vi "backup_imp_test_v4.vi"() -> ()   [LabVIEW 2014]
uses:
  <vilib>/LabVIEW Targets/FPGA/cRIO/shared/nicrio_ModuleControls/nicrio_cRIO-9237_DataRatesRing.ctl
  <vilib>/LabVIEW Targets/FPGA/cRIO/shared/nicrio_ModuleControls/nicrio_cRIO-9237_ExcitationVoltageRing.ctl
  <vilib>/rvi/FXPMathLib/FxpSinAndCos/subVIs/nifxpmath_SinAndCos_SimConfig.ctl
  <vilib>/rvi/Emulation/niFpgaGetClockAttributes.vi
  <vilib>/rvi/Emulation/niFpgaSctlEmulationGetInTimedLoop.vi
  <vilib>/rvi/Emulation/niFpgaEmulationReportErrorSimple.vi
  <vilib>/rvi/Emulation/niFpgaProcessEmulError.vi
  <vilib>/rvi/interface/RandomDataEmulation/nirviRandomDataMultiElementFPGAFIFO.vi
  <instcachedir>/0/nirviRandomDataMultiElementFPGAFIFO_AD0CFC12EF974623A9C2E4184BC062B2.lvgen/nirviRandomDataMultiElementFPGAFIFO_AD0CFC12EF974623A9C2E4184BC062B2_023.vi
  <vilib>/rvi/interface/RandomDataEmulation/niFpgaRandomDataHandleErrors.vi
  <vilib>/rvi/Emulation/niFpgaCriticalErrorInLSC.vi
  <vilib>/rvi/eio/common/nirviEmuTemplateMethod_errors.vi
  <vilib>/rvi/FXPMathLib/FxpSinAndCos/simVIs/DllFxpSinAndCosTemp_sub.vi
  <vilib>/rvi/eio/common/nirviEmuTemplatePropertySet_errors.vi
  <vilib>/rvi/DataTransferAndStorage/Container/XNode/niFpgaContainer.xnode
  <vilib>/rvi/interface/RandomDataEmulation/nirviRandomDataFpgaMultiElementTemplate.vi
  <vilib>/eio/EIONode/EIONode.xnode
  <vilib>/rvi/FXPMathLib/FxpMul/XNode/nifxpmath_Multiplier.xnode
  <vilib>/rvi/FXPMathLib/FxpSinAndCos/XNode/nifxpmath_SinAndCos.xnode
  <vilib>/rvi/Analysis/measure/butterworth/XNode/niFpgaButterworthFilter.xnode
  <vilib>/rvi/FXPMathLib/FxpSub/XNode/nifxpmath_Sub.xnode
  <vilib>/rvi/FXPMathLib/FxpAdd/XNode/nifxpmath_Add.xnode
  <vilib>/eio/EIOPropertyNode/EIOPropertyNode.xnode
  <vilib>/rvi/eio/common/nirviEmuTemplatePropertyGet_errors.vi
  <vilib>/rvi/eio/common/nirviEmuTemplatePropertyGet_noerrors.vi
  <vilib>/rvi/eio/common/nirviEmuTemplatePropertySet_noerrors.vi
  <vilib>/rvi/FXPMathLib/sim/FxpSim.dll
panel:
  out "Fp_dc":fxp<+/-,32,10>
  out "Fy_dc":fxp<+/-,32,10>
  in  "Zero_y":bool
  in  "Zero_p":bool
  in  "mt0_omega_p":u32
  in  "Encoder reset":bool
  out "fpt_d":fxp<+/-,36,18>
  out "Dp_error_dd":fxp<+/-,36,16>
  out "Dp_error_d":fxp<+/-,33,8>
  in  "Dp_dd coeff.":i32[](array[numeric])=[946630756, 63555534]
  out "Dp_dd":fxp<+/-,36,25>
  out "dFp_PID":fxp<+/-,36,18>
  in  "dFp_PID coeff.":i32[](array[numeric])=[946630756, 63555534]
  out "fpt_i":fxp<+/-,34,18>
  in  "Bv_p":fxp<+/-,22,8>
  in  "Kv_p":fxp<+/-,22,8>
  out "Dp_error":fxp<+/-,22,7>
  out "Dpr_sin":fxp<+/-,22,7>
  in  "Sin offset_p":fxp<+/-,22,7>
  in  "Sin magnitude_p":fxp<+/-,21,6>
  out "Dpr_sin_dd":fxp<+/-,35,20>
  out "Dpr_sin_d":fxp<+/-,33,15>
  out "Sin omega_p":fxp<+/-,34,9>
  in  "Sin wave freq._p (Hz)":fxp<+/-,32,6>
  in  "Dpr_step":fxp<+/-,22,7>
  out "Dpr_for":fxp<+/-,22,7>
  in  "Command_p":i16(ring) items=["Step", "Sine"]
  in  "Ki_p":fxp<+/-,36,9>
  out "Fp_PID":fxp<+/-,36,16>
  in  "fp_tolorance":fxp<+,22,6>
  out "fp_tilde":fxp<+/-,33,10>
  in  "Kd_p":fxp<+/-,36,9>
  in  "Kp_p":fxp<+/-,36,9>
  out "Fr_p":fxp<+/-,32,10>
  in  "S/F coeff_p":fxp<+/-,25,-10>
  in  "S/F coeff_y":fxp<+/-,25,-10>
  out "va_p":fxp<+/-,36,7>
  out "vb_p":fxp<+/-,37,8>
  out "vq_p_F":fxp<+/-,20,5> format="%.57g"
  out "vd_p_F":fxp<+/-,20,5>
  in  "dFp_add":bool
  in  "Stop motor_p":bool
  out "Force_p":fxp<+/-,32,10>
  in  "Strain selection_p":i16(ring) items=["Raw", "Avg.", "Avg. w. filter"]
  out "Strain_p (Avg w. f)":fxp<+/-,36,8>
  in  "Strain_p mean coeff.":i32[](array[numeric])=[946630756, 63555534]
  out "Strain_p (Avg)":fxp<+/-,32,4>
  out "Raw Strain_p":fxp<+/-,36,4>
  out "Mod6/AI3":fxp<+/-,32,4>
  in  "Strain gage reset_p":bool
  out "Dp_d (mm/s)":fxp<+/-,36,11>
  out "omega_p (rad/s)":fxp<+/-,20,9>
  out "mt_omega_p":u32
  out "rad_p(NrTheta)":fxp<+/-,33,20>
  out "D_p(mm)":fxp<+/-,32,7>
  out "Encoder Position_p":i32
  in  "Encoder reset_p":bool
  out "Strain_y (Avg w. f)":fxp<+/-,36,8>
  in  "Strain_y mean coeff.":i32[](array[numeric])=[-898916953, 1957103773, 3888751]
  out "Dyr_for":fxp<+/-,22,7>
  in  "Command_y":i16(ring) items=["Step", "Sine"]
  out "Strain_y (Avg)":fxp<+/-,32,4>
  in  "Strain selection_y":i16(ring) items=["Raw", "Avg.", "Avg. w. filter"]
  out "vb_y":fxp<+/-,38,8>
  out "va_y":fxp<+/-,38,8>
  out "fyt_d":fxp<+/-,36,18>
  out "Fr_y":fxp<+/-,32,10>
  in  "Bv_y":fxp<+/-,22,8>
  out "Dy_error_dd":fxp<+/-,36,16>
  out "Dy_error_d":fxp<+/-,33,8>
  in  "Kv_y":fxp<+/-,22,8>
  out "Dy_error":fxp<+/-,22,7>
  out "Dyr_sin_dd":fxp<+/-,35,20>
  out "Dyr_sin_d":fxp<+/-,33,15>
  out "Sin omega_y":fxp<+/-,34,9>
  out "Dyr_sin":fxp<+/-,22,7>
  in  "Sin offset_y":fxp<+/-,22,7>
  in  "Sin magnitude_y":fxp<+/-,21,6>
  out "Time now(s)":fxp<+,52,14>
  in  "Sin wave freq._y (Hz)":fxp<+/-,32,6>
  in  "Dyr_step":fxp<+/-,22,7>
  in  "Drive mode":i16(ring) items=["Backward", "Forward"]
  out "Dy_dd":fxp<+/-,36,25>
  in  "Dy_dd coeff.":i32[](array[numeric])=[946630756, 63555534]
  out "dFy_PID":fxp<+/-,36,18>
  in  "dFy_PID coeff.":i32[](array[numeric])=[946630756, 63555534]
  out "fyt_i":fxp<+/-,36,16>
  out "Fy_PID":fxp<+/-,36,16>
  in  "fy_tolorance":fxp<+,22,6>
  in  "Ki_y":fxp<+/-,36,9>
  in  "Kd_y":fxp<+/-,36,9>
  out "fy_tilde":fxp<+/-,32,10>
  in  "Kp_y":fxp<+/-,36,9>
  out "vq_y_F":fxp<+/-,20,5> format="%.57g"
  out "vd_y_F":fxp<+/-,20,5>
  in  "dFy_add":bool
  in  "Stop motor_y":bool
  out "Dy_d (mm/s)":fxp<+/-,36,11>
  out "omega_y (rad/s)":fxp<+/-,20,9>
  in  "mt0_omega_y":u32
  out "mt_omega_y":u32
  out "rad_y(NrTheta)":fxp<+/-,33,20>
  out "D_y(mm)":fxp<+/-,32,7>
  out "Encoder Position_y":i32
  in  "Encoder reset_y":bool
  in  "Ini coe.":bool
  out "Loop rate (kHz)":fxp<+/-,36,7>
  out "Force_y":fxp<+/-,32,10>
  out "Raw Strain_y":fxp<+/-,36,4>
  in  "Strain gage reset_y":bool
  in  "Stop (Strain)":bool
  out "Mod6/AI2":fxp<+/-,32,4>
  in  "Excitation Voltage":T1 items=["2.5 Volts", "3.3 Volts", "5.0 Volts", "10.0 Volts", "External Excitation"]
  in  "Data Rate":T2=1 items=["50.000 kS/s (NI 9237)"=1, "25.000 kS/s (NI 9237)"=2, "16.667 kS/s (NI 9237)"=3, "12.500 kS/s (NI 9237)"=4, "10.000 kS/s (NI 9237)"=5, "8.333 kS/s (NI 9237)"=6, "7.143 kS/s (NI 9237)"=7, "6.250 kS/s (NI 9237)"=8, "5.556 kS/s (NI 9237)"=9, "5.000 kS/s (NI 9237)"=10, "4.545 kS/s (NI 9237)"=11, "4.167 kS/s (NI 9237)"=12, "3.846 kS/s (NI 9237)"=13, "3.571 kS/s (NI 9237)"=14, "3.333 kS/s (NI 9237)"=15, "3.125 kS/s (NI 9237)"=16, "2.941 kS/s (NI 9237)"=17, "2.778 kS/s (NI 9237)"=18, "2.632 kS/s (NI 9237)"=19, "2.500 kS/s (NI 9237)"=20, "2.381 kS/s (NI 9237)"=21, "2.273 kS/s (NI 9237)"=22, "2.174 kS/s (NI 9237)"=23, "2.083 kS/s (NI 9237)"=24, "2.000 kS/s (NI 9237)"=25, "1.923 kS/s (NI 9237)"=26, "1.852 kS/s (NI 9237)"=27, "1.786 kS/s (NI 9237)"=28, "1.724 kS/s (NI 9237)"=29, "1.667 kS/s (NI 9237)"=30, "1.613 kS/s (NI 9237)"=31]
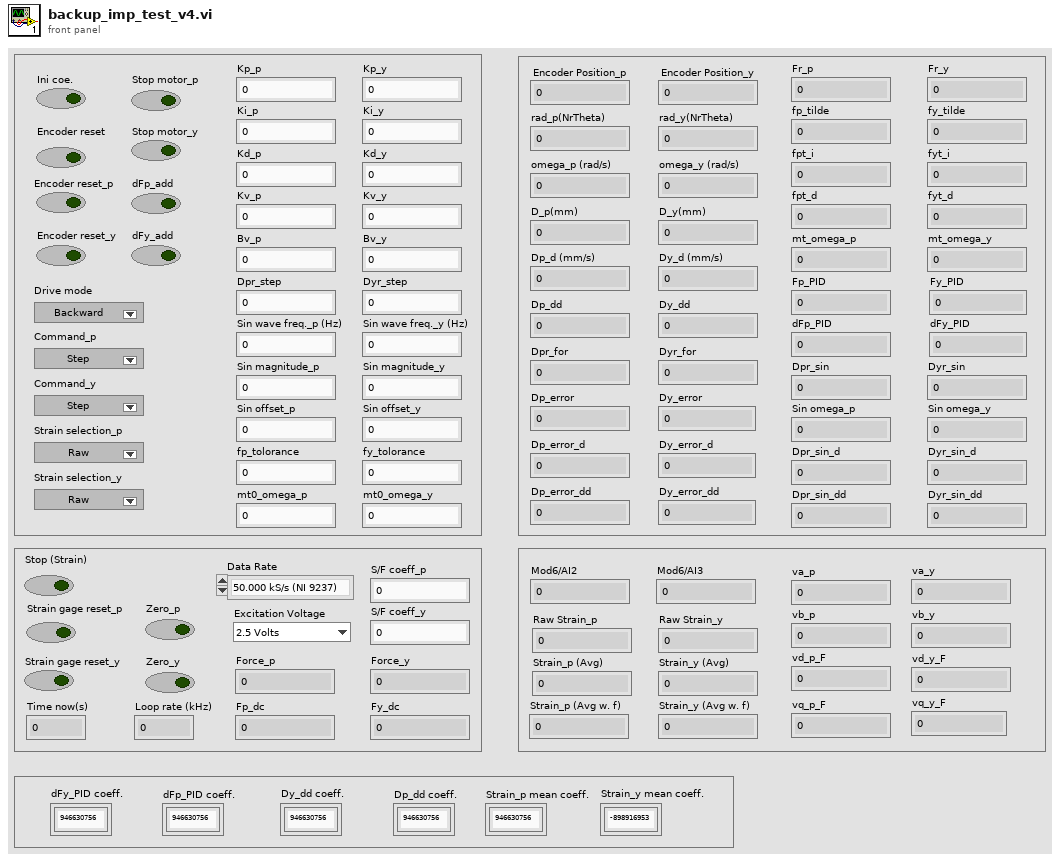
[diagram p1: front panel]
types:
  T1 = typedef "nicrio_cRIO-9237_ExcitationVoltageRing.ctl" = u8
  T2 = typedef "nicrio_cRIO-9237_DataRatesRing.ctl" = u8
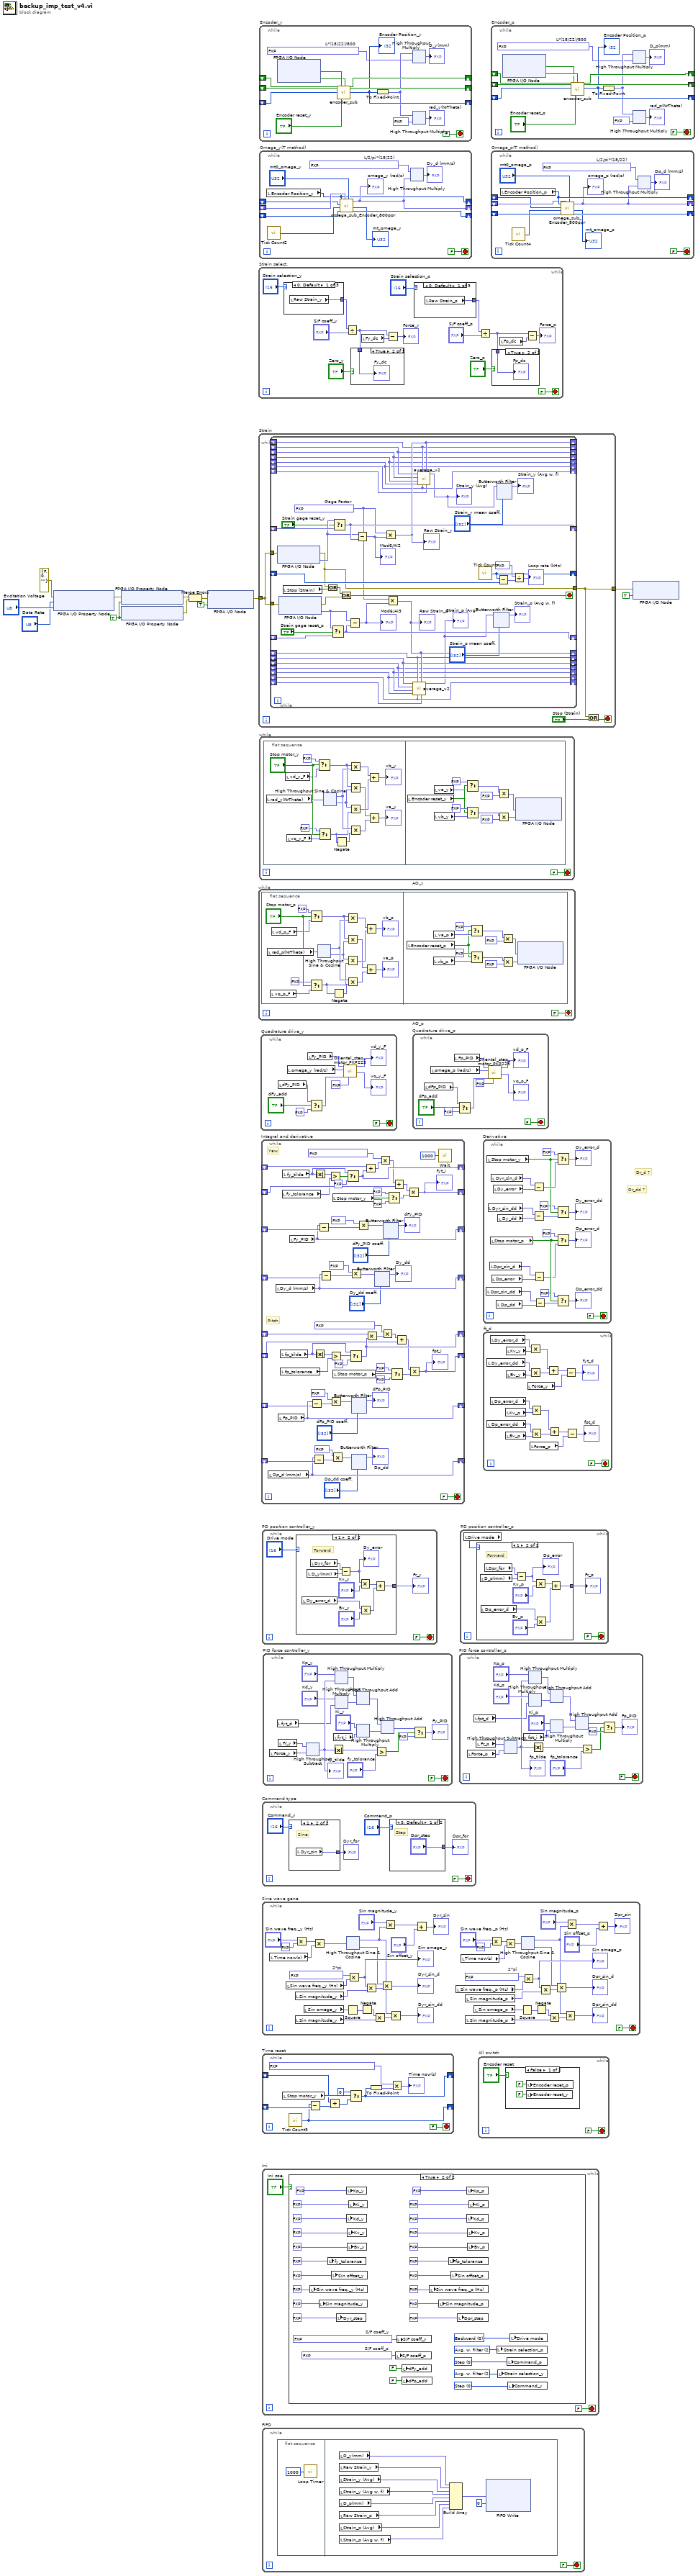
[diagram p0: block diagram]
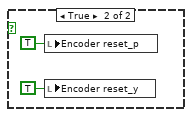
[diagram p2: hidden frame]
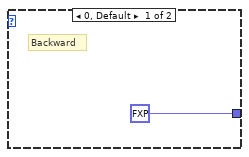
[diagram p3: hidden frame]
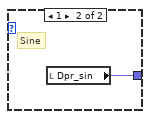
[diagram p4: hidden frame]
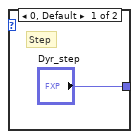
[diagram p5: hidden frame]
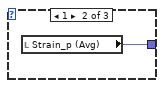
[diagram p8: hidden frame]
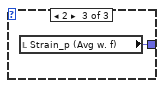
[diagram p9: hidden frame]
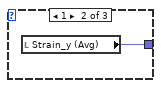
[diagram p10: hidden frame]
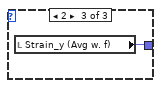
[diagram p11: hidden frame]
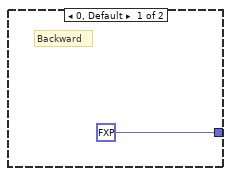
[diagram p12: hidden frame]
diagram:
  w5 = TRUE ("Half-Bridge Enable")
  # "Dr_dd ?"
  # "Dr_d ?"
  n1 = xnode "FPGA I/O Property Node"("error in"=errorcluster {"status"=FALSE, "code"=0, "source"=""}, "Data Rate"="Data Rate", "Excitation Voltage"="Excitation Voltage") -> ("error out"=w10:errorcluster)  [unwired: 1 in, 1 out]
  n2 = xnode "FPGA I/O Property Node"("error in"=w10, "Half-Bridge Enable"=w5) -> ("error out"=w3:errorcluster)  [unwired: 1 in, 1 out]
  n3 = xnode "FPGA I/O Property Node"("Half-Bridge Enable"=w5) -> ("error out"=w2:errorcluster)  [unwired: 2 in, 1 out]
  n4 = Merge Errors(w3, w2) -> (w4:errorcluster)
  n5 = xnode "FPGA I/O Node"("error in"=w4, "Mod6/Start"=TRUE) -> ("error out"=w8:errorcluster)  [unwired: 1 in, 1 out]
  n6 = while "Strain select." {
    stop <- FALSE stop-if-true
    n7 = case shown="0, Default" "Strain selection_y" {
      tunnel: [w33 w34 w35] -> w26
      frame 0, Default {
        n8 = local read "Raw Strain_y"() -> (w33:fxp<+/-,36,4>)
      }
      frame 1 {
        n9 = local read "Strain_y (Avg)"() -> (w34:fxp<+/-,32,4>)
      }
      frame 2 {
        n10 = local read "Strain_y (Avg w. f)"() -> (w35:fxp<+/-,36,8>)
      }
    }
    n11 = Divide(x=w26, y="S/F coeff_y") -> (x/y=w19:fxp<+/-,32,10>)
    n12 = case shown="True" "Zero_y" {
      tunnel: w19 -> [_ w29]
      frame False {
      }
      frame True {
        "Fy_dc" <- w29
      }
    }
    n13 = local read "Fy_dc"() -> (w20:fxp<+/-,32,10>)
    n14 = Subtract(x=w19, y=w20) -> (x-y=→"Force_y":fxp<+/-,33,11>)
    n15 = case shown="0, Default" "Strain selection_p" {
      tunnel: [w30 w31 w32] -> w24
      frame 0, Default {
        n16 = local read "Raw Strain_p"() -> (w30:fxp<+/-,36,4>)
      }
      frame 1 {
        n17 = local read "Strain_p (Avg)"() -> (w31:fxp<+/-,32,4>)
      }
      frame 2 {
        n18 = local read "Strain_p (Avg w. f)"() -> (w32:fxp<+/-,36,8>)
      }
    }
    n19 = Divide(x=w24, y="S/F coeff_p") -> (x/y=w16:fxp<+/-,32,10>)
    n20 = case shown="True" "Zero_p" {
      tunnel: w16 -> [_ w28]
      frame False {
      }
      frame True {
        "Fp_dc" <- w28
      }
    }
    n21 = local read "Fp_dc"() -> (w14:fxp<+/-,32,10>)
    n22 = Subtract(x=w16, y=w14) -> (x-y=→"Force_p":fxp<+/-,33,11>)
  }
  n23 = while "Strain" {
    tunnel: w8 -> [w38]
    tunnel: [w36] -> w1
    stop <- w37 stop-if-true
    n24 = while {
      tunnel: w38 -> [w84]
      tunnel: [w57] -> w36
      shift-right: [w81] -> _
      shift-left: _ -> [w82]
      shift-right: [w77] -> _
      shift-left: _ -> [w78]
      shift-right: [w72] -> _
      shift-left: _ -> [w71]
      shift-right: [w71] -> _
      shift-left: _ -> [w70]
      shift-right: [w70] -> _
      shift-left: _ -> [w69]
      shift-right: [w69] -> _
      shift-left: _ -> [w68]
      shift-right: [w68] -> _
      shift-left: _ -> [w67]
      shift-right: [w67] -> _
      shift-left: _ -> [w66]
      shift-right: [w66] -> _
      shift-left: _ -> [w65]
      tunnel: w38 -> [w61]
      shift-right: [w54] -> _
      shift-left: _ -> [w55]
      shift-right: [w50] -> _
      shift-left: _ -> [w49]
      shift-right: [w49] -> _
      shift-left: _ -> [w48]
      shift-right: [w48] -> _
      shift-left: _ -> [w47]
      shift-right: [w47] -> _
      shift-left: _ -> [w46]
      shift-right: [w46] -> _
      shift-left: _ -> [w45]
      shift-right: [w45] -> _
      shift-left: _ -> [w44]
      shift-right: [w44] -> _
      shift-left: _ -> [w43]
      stop <- w58 stop-if-true
      w52 = fxp<+,20,2> 2.115001678466797  # Gage Factor
      n25 = xnode "FPGA I/O Node"("error in"=w84) -> ("error out"=w57:errorcluster, "Mod6/AI2"=w79:fxp<+/-,24,-4>)  [unwired: 1 in, 1 out]
      n26 = xnode "FPGA I/O Node"("error in"=w61) -> ("error out"=w59:errorcluster, "Mod6/AI3"=w53:fxp<+/-,24,-4>)  [unwired: 1 in, 1 out]
      n27 = local read "Stop (Strain)"() -> (w83:bool)
      n28 = Or(x=w57, y=w83) -> (x .or. y?=w60:bool)
      n29 = Select(t=w53, s="Strain gage reset_p", f=w55) -> (s? t:f=w54:fxp<+/-,24,-4>)
      n30 = Select(t=w79, s="Strain gage reset_y", f=w82) -> (s? t:f=w81:fxp<+/-,24,-4>)
      n31 = Or(x=w60, y=w59) -> (x .or. y?=w58:bool)
      n32 = Subtract(x=w53, y=w54) -> (x-y=w51:fxp<+/-,25,-3>)
      "Mod6/AI3" <- w51
      n33 = Subtract(x=w79, y=w81) -> (x-y=w80:fxp<+/-,25,-3>)
      "Mod6/AI2" <- w80
      n34 = Multiply(x=w52, y=w80) -> (x*y=w72:fxp<+/-,41,6>)
      "Raw Strain_y" <- w72
      n35 = Multiply(x=w52, y=w51) -> (x*y=w50:fxp<+/-,45,-1>)
      "Raw Strain_p" <- w50
      n36 = call "average_v2.vi"("Numeric 8"=w43, "Numeric"=w50, "Numeric 7"=w44, "Numeric 2"=w49, "Numeric 6"=w45, "Numeric 5"=w46, "Numeric 4"=w47, "Numeric 3"=w48) -> ("Mean (8pt)"=w42:fxp<+/-,32,4>)  [unwired: 1 in, 2 out]
      "Strain_p (Avg)" <- w42
      n37 = call "average_v2.vi"("Numeric 8"=w65, "Numeric"=w72, "Numeric 7"=w66, "Numeric 2"=w71, "Numeric 6"=w67, "Numeric 5"=w68, "Numeric 4"=w69, "Numeric 3"=w70) -> ("Mean (8pt)"=w64:fxp<+/-,32,4>)  [unwired: 1 in, 2 out]
      "Strain_y (Avg)" <- w64
      n38 = call "Tick Count"() -> ("Tick Count(uSec)"=w77:u32)
      n39 = xnode "Butterworth Filter"("input data"=w42, "scaled coefficients"="Strain_p mean coeff.") -> ("output data"=→"Strain_p (Avg w. f)":fxp<+/-,36,8>)  [unwired: 1 in]
      n40 = xnode "Butterworth Filter"("input data"=w64, "scaled coefficients"="Strain_y mean coeff.") -> ("output data"=→"Strain_y (Avg w. f)":fxp<+/-,32,4>)  [unwired: 1 in]
      n41 = Subtract(x=w77, y=w78) -> (x-y=w75:fxp<+/-,32,16>)
      n42 = Divide(x=fxp<+,7,10> 1000.0, y=w75) -> (x/y=→"Loop rate (kHz)":fxp<+/-,40,27>)
    }
    n43 = Or(x=w36, y="Stop (Strain)") -> (x .or. y?=w37:bool)
  }
  n44 = while "AO_p" {
    stop <- FALSE stop-if-true
    n45 = flat-sequence {
      frame #0 {
        n46 = local read "rad_p(NrTheta)"() -> (w113:fxp<+/-,33,20>)
        n47 = local read "vq_p_F"() -> (w114:fxp<+/-,20,5>)
        n48 = local read "vd_p_F"() -> (w116:fxp<+/-,20,5>)
        n49 = Select(t=fxp<+/-,20,5> 0.0, s="Stop motor_p", f=w116) -> (s? t:f=w105:fxp<+/-,20,5>)
        n50 = Select(t=fxp<+,1,1> 0.0, s="Stop motor_p", f=w114) -> (s? t:f=w104:fxp<+/-,20,5>)
        n51 = xnode "High Throughput Sine & Cosine"("x (pi)"=w113) -> ("sin(x)"=w107:fxp<+/-,16,2>, "cos(x)"=w106:fxp<+/-,16,2>)
        n52 = Negate(x=w104) -> (-x=w112:fxp<+/-,21,6>)
        n53 = Multiply(x=w105, y=w107) -> (x*y=w111:fxp<+/-,36,7>)
        n54 = Multiply(x=w105, y=w106) -> (x*y=w109:fxp<+/-,36,7>)
        n55 = Multiply(x=w106, y=w104) -> (x*y=w110:fxp<+/-,36,7>)
        n56 = Multiply(x=w107, y=w112) -> (x*y=w108:fxp<+/-,35,6>)
        n57 = Add(x=w111, y=w110) -> (x+y=→"vb_p":fxp<+/-,37,8>)
        n58 = Add(x=w109, y=w108) -> (x+y=→"va_p":fxp<+/-,36,7>)
      }
      frame #1 {
        n59 = local read "Encoder reset_p"() -> (w149:bool)
        n60 = local read "vb_p"() -> (w150:fxp<+/-,37,8>)
        n61 = local read "va_p"() -> (w151:fxp<+/-,36,7>)
        n62 = Select(t=fxp<+,2,2> 3.0, s=w149, f=w151) -> (s? t:f=w157:fxp<+/-,36,7>)
        n63 = Select(t=fxp<+,1,1> 0.0, s=w149, f=w150) -> (s? t:f=w156:fxp<+/-,37,8>)
        n64 = Multiply(x=w157, y=fxp<+/-,1,0> -0.5) -> (x*y=w152:fxp<+/-,36,6>)
        n65 = Multiply(x=w156, y=fxp<+/-,1,0> -0.5) -> (x*y=w153:fxp<+/-,36,6>)
        n66 = xnode "FPGA I/O Node"("Mod8/AO0"=w152, "Mod8/AO1"=w153) -> ()  [unwired: 2 in, 2 out]
      }
    }
  }
  n67 = while "AO_y" {
    stop <- FALSE stop-if-true
    n68 = flat-sequence {
      frame #0 {
        n69 = local read "rad_y(NrTheta)"() -> (w177:fxp<+/-,33,20>)
        n70 = local read "vd_y_F"() -> (w175:fxp<+/-,20,5>)
        n71 = local read "vq_y_F"() -> (w174:fxp<+/-,20,5>)
        n72 = Select(t=fxp<+/-,20,5> 0.0, s="Stop motor_y", f=w175) -> (s? t:f=w169:fxp<+/-,20,5>)
        n73 = Select(t=fxp<+/-,20,5> 0.0, s="Stop motor_y", f=w174) -> (s? t:f=w168:fxp<+/-,20,5>)
        n74 = xnode "High Throughput Sine & Cosine"("x (pi)"=w177) -> ("sin(x)"=w171:fxp<+/-,17,2>, "cos(x)"=w170:fxp<+/-,17,2>)
        n75 = Negate(x=w168) -> (-x=w167:fxp<+/-,21,6>)
        n76 = Multiply(x=w169, y=w171) -> (x*y=w166:fxp<+/-,37,7>)
        n77 = Multiply(x=w169, y=w170) -> (x*y=w164:fxp<+/-,37,7>)
        n78 = Multiply(x=w170, y=w168) -> (x*y=w165:fxp<+/-,37,7>)
        n79 = Multiply(x=w171, y=w167) -> (x*y=w163:fxp<+/-,36,6>)
        n80 = Add(x=w166, y=w165) -> (x+y=→"vb_y":fxp<+/-,38,8>)
        n81 = Add(x=w164, y=w163) -> (x+y=→"va_y":fxp<+/-,37,7>)
      }
      frame #1 {
        n82 = local read "Encoder reset_y"() -> (w210:bool)
        n83 = local read "va_y"() -> (w209:fxp<+/-,38,8>)
        n84 = local read "vb_y"() -> (w208:fxp<+/-,38,8>)
        n85 = Select(t=fxp<+,2,2> 3.0, s=w210, f=w209) -> (s? t:f=w214:fxp<+/-,38,8>)
        n86 = Select(t=fxp<+,1,1> 0.0, s=w210, f=w208) -> (s? t:f=w213:fxp<+/-,38,8>)
        n87 = Multiply(x=w214, y=fxp<+/-,1,0> -0.5) -> (x*y=w217:fxp<+/-,39,8>)
        n88 = Multiply(x=w213, y=fxp<+/-,1,0> -0.5) -> (x*y=w218:fxp<+/-,37,6>)
        n89 = xnode "FPGA I/O Node"("Mod8/AO2"=w217, "Mod8/AO3"=w218) -> ()  [unwired: 2 in, 2 out]
      }
    }
  }
  n90 = while "Encoder_y" {
    shift-right: [w230] -> _
    shift-left: _ -> [w231]
    shift-right: [w232] -> _
    shift-left: _ -> [w233]
    shift-right: [w225] -> _
    shift-left: _ -> [w229]
    stop <- FALSE stop-if-true
    w222 = fxp<+/-,32,0> 0.0020454544574022293  # L*(18/22)/800
    n91 = xnode "FPGA I/O Node"() -> ("Mod4/DI3"=w228:bool, "Mod4/DI4"=w227:bool)  [unwired: 2 in, 2 out]
    n92 = call "encoder_sub.vi"("A_pre"=w231, "B_pre"=w233, "Encoder Position_pre"=w229, "A input"=w228, "Encoder Position Reset"="Encoder reset_y", "B input"=w227) -> ("A"=w230:bool, "B"=w232:bool, "Encoder Position (Counts)"=w225:i32)  [unwired: 19 in]
    "Encoder Position_y" <- w225
    n93 = To Fixed-Point(number=w225) -> (fixed-point=w224:fxp<+/-,32,32>)  [unwired: 1 in]
    n94 = xnode ("High Throughput Multiply")("x"=w224, "y"=w222) -> ("x*y"=→"D_y(mm)":fxp<+/-,64,32>)
    n95 = xnode ("High Throughput Multiply")("x"=w224, "y"=fxp<+/-,16,1> 0.125) -> ("x*y"=→"rad_y(NrTheta)":fxp<+/-,48,33>)
  }
  n96 = while "Omega_y(T method)" {
    shift-right: [w235] -> _
    shift-left: _ -> [w236]
    shift-right: [w239] -> _
    shift-left: _ -> [w241]
    shift-right: [w243] -> _
    shift-left: _ -> [w244]
    stop <- FALSE stop-if-true
    w238 = fxp<+/-,32,0> 0.2604353614151478  # L/2/pi*(18/22)
    n97 = local read "Encoder Position_y"() -> (w235:i32)
    n98 = call "Tick Count2"() -> ("Tick Count(Ticks)"=w245:u32)
    n99 = call "omega_sub_Encoder_800ppr.vi"("mt0"="mt0_omega_y", "omega_pre"=w241, "ticks_m_pre"=w244, "ticks"=w245, "count_pre"=w236, "count"=w235) -> ("ticks_m"=w243:u32, "mt"=→"mt_omega_y":u32, "omega"=w239:fxp<+/-,36,13>)  [unwired: 3 in]
    "omega_y (rad/s)" <- w239
    n100 = xnode ("High Throughput Multiply")("x"=w238, "y"=w239) -> ("x*y"=→"Dy_d (mm/s)":fxp<+/-,64,13>)
  }
  n101 = while "Quadrature drive_y" {
    stop <- FALSE stop-if-true
    n102 = local read "dFy_PID"() -> (w247:fxp<+/-,36,18>)
    n103 = local read "omega_y (rad/s)"() -> (w255:fxp<+/-,20,9>)
    n104 = local read "Fy_PID"() -> (w248:fxp<+/-,36,16>)
    n105 = Select(t=w247, s="dFy_add", f=fxp<+,1,1> 0.0) -> (s? t:f=w251:fxp<+/-,36,18>)
    n106 = call "Oriental_step_motor_PKP225.vi"("F_Threshold"=fxp<+,12,12> 10.0, "dFmr"=w251, "omega"=w255, "Fmr"=w248) -> ("vq_F"=→"vq_y_F":fxp<+/-,20,5>, "vd_F"=→"vd_y_F":fxp<+/-,20,5>)  [unwired: 6 in]
  }
  n107 = while "Integral and derivative" {
    shift-right: [w311] -> _
    shift-left: _ -> [w310]
    shift-right: [w303] -> _
    shift-left: _ -> [w302]
    shift-right: [w313] -> _
    shift-left: _ -> [w314]
    shift-right: [w293] -> _
    shift-left: _ -> [w292]
    shift-right: [w279] -> _
    shift-left: _ -> [w282]
    shift-right: [w272] -> _
    shift-left: _ -> [w271]
    shift-right: [w266] -> _
    shift-left: _ -> [w265]
    shift-right: [w261] -> _
    shift-left: _ -> [w262]
    stop <- FALSE stop-if-true
    # "Pitch"
    # "Yaw"
    n108 = local read "Dp_d (mm/s)"() -> (w261:fxp<+/-,36,11>)
    n109 = local read "Dy_d (mm/s)"() -> (w293:fxp<+/-,36,11>)
    n110 = local read "Fp_PID"() -> (w266:fxp<+/-,36,16>)
    n111 = local read "fp_tilde"() -> (w283:fxp<+/-,33,10>)
    n112 = local read "fp_tolorance"() -> (w286:fxp<+,22,6>)
    n113 = local read "fy_tolorance"() -> (w289:fxp<+,22,6>)
    n114 = local read "fy_tilde"() -> (w315:fxp<+/-,32,10>)
    n115 = local read "Fy_PID"() -> (w313:fxp<+/-,36,16>)
    n116 = Subtract(x=w266, y=w265) -> (x-y=w270:fxp<+/-,37,17>)
    n117 = Subtract(x=w261, y=w262) -> (x-y=w263:fxp<+/-,37,12>)
    n118 = Absolute Value(x=w283) -> (abs(x)=w287:fxp<+,33,10>)
    n119 = Absolute Value(x=w315) -> (abs(x)=w317:fxp<+,32,10>)
    n120 = Subtract(x=w313, y=w314) -> (x-y=w301:fxp<+/-,37,17>)
    n121 = Subtract(x=w293, y=w292) -> (x-y=w295:fxp<+/-,36,11>)
    n122 = Greater?(x=w317, y=w289) -> (0:w318:bool)
    n123 = Greater?(x=w287, y=w286) -> (0:w285:bool)
    n124 = Multiply(x=fxp<+,7,10> 1000.0, y=w270) -> (x*y=w268:fxp<+/-,32,18>)
    n125 = Multiply(x=fxp<+,7,10> 1000.0, y=w263) -> (x*y=w259:fxp<+/-,36,21>)
    n126 = local read "Stop motor_y"() -> (w304:bool)
    n127 = local read "Stop motor_p"() -> (w274:bool)
    n128 = Select(t=w315, s=w318, f=fxp<+/-,33,11> 0.0) -> (s? t:f=w311:fxp<+/-,33,11>)
    n129 = Select(t=w283, s=w285, f=fxp<+,1,1> 0.0) -> (s? t:f=w279:fxp<+/-,33,10>)
    n130 = Multiply(x=fxp<+,7,10> 1000.0, y=w295) -> (x*y=w294:fxp<+/-,36,21>)
    n131 = xnode "Butterworth Filter"("input data"=w268, "scaled coefficients"="dFp_PID coeff.") -> ("output data"=→"dFp_PID":fxp<+/-,36,22>)  [unwired: 1 in]
    n132 = xnode "Butterworth Filter"("input data"=w259, "scaled coefficients"="Dp_dd coeff.") -> ("output data"=→"Dp_dd":fxp<+/-,36,25>)  [unwired: 1 in]
    n133 = Multiply(x=fxp<+,7,10> 1000.0, y=w301) -> (x*y=w298:fxp<+/-,32,18>)
    n134 = Add(x=w310, y=w311) -> (x+y=w316:fxp<+/-,34,12>)
    n135 = Multiply(x=w282, y=w279) -> (x*y=w281:fxp<+/-,34,12>)
    n136 = xnode "Butterworth Filter"("input data"=w294, "scaled coefficients"="Dy_dd coeff.") -> ("output data"=→"Dy_dd":fxp<+/-,36,25>)  [unwired: 1 in]
    n137 = Multiply(x=fxp<+/-,30,12> 0.000499725341796875, y=w316) -> (x*y=w309:fxp<+/-,34,10>)
    n138 = Multiply(x=fxp<+/-,30,12> 0.000499725341796875, y=w281) -> (x*y=w278:fxp<+/-,34,10>)
    n139 = xnode "Butterworth Filter"("input data"=w298, "scaled coefficients"="dFy_PID coeff.") -> ("output data"=→"dFy_PID":fxp<+/-,36,22>)  [unwired: 1 in]
    n140 = Select(t=fxp<+,1,1> 0.0, s=w304, f=fxp<+,1,1> 1.0) -> (s? t:f=w307:fxp<+,1,1>)
    n141 = Select(t=fxp<+,1,1> 0.0, s=w274, f=fxp<+,1,1> 1.0) -> (s? t:f=w276:fxp<+,1,1>)
    n142 = Add(x=w309, y=w302) -> (x+y=w308:fxp<+/-,36,16>)
    n143 = Add(x=w278, y=w271) -> (x+y=w277:fxp<+/-,36,16>)
    n144 = Multiply(x=w308, y=w307) -> (x*y=w303:fxp<+/-,34,18>)
    "fyt_i" <- w303
    n145 = Multiply(x=w277, y=w276) -> (x*y=w272:fxp<+/-,34,18>)
    "fpt_i" <- w272
    n146 = call "Wait"("Count(uSec)"=u32 1000) -> ()  [unwired: 1 out]
  }
  n147 = while "PD position controller_y" {
    stop <- FALSE stop-if-true
    n148 = case shown="1" "Drive mode" {
      tunnel: [fxp<+/-,62,19> 0.0 w357] -> w353
      frame 0, Default {
        # "Backward"
      }
      frame 1 {
        # "Forward"
        n149 = local read "Dy_error_d"() -> (w359:fxp<+/-,33,8>)
        n150 = local read "D_y(mm)"() -> (w364:fxp<+/-,32,7>)
        n151 = local read "Dyr_for"() -> (w356:fxp<+/-,22,7>)
        n152 = Subtract(x=w356, y=w364) -> (x-y=w363:fxp<+/-,33,8>)
        "Dy_error" <- w363
        n153 = Multiply(x=w363, y="Kv_y") -> (x*y=w361:fxp<+/-,54,15>)
        n154 = Multiply(x=w359, y="Bv_y") -> (x*y=w358:fxp<+/-,55,16>)
        n155 = Add(x=w361, y=w358) -> (x+y=w357:fxp<+/-,55,16>)
      }
    }
    "Fr_y" <- w353
  }
  n156 = while "Command type" {
    stop <- FALSE stop-if-true
    n157 = case shown="1" "Command_y" {
      tunnel: ["Dyr_step" w373] -> w368
      frame 0, Default {
        # "Step"
      }
      frame 1 {
        # "Sine"
        n158 = local read "Dyr_sin"() -> (w373:fxp<+/-,22,7>)
      }
    }
    "Dyr_for" <- w368
    n159 = case shown="0, Default" "Command_p" {
      tunnel: ["Dpr_step" w371] -> w366
      frame 0, Default {
        # "Step"
      }
      frame 1 {
        # "Sine"
        n160 = local read "Dpr_sin"() -> (w371:fxp<+/-,22,7>)
      }
    }
    "Dpr_for" <- w366
  }
  n161 = while "Sine wave gene" {
    stop <- FALSE stop-if-true
    w379 = fxp<+,20,3> 6.2831878662109375  # 2*pi
    w411 = fxp<+,20,3> 6.2831878662109375  # 2*pi
    n162 = local read "Time now(s)"() -> (w417:fxp<+,52,14>)
    n163 = local read "Sin wave freq._y (Hz)"() -> (w410:fxp<+/-,32,6>)
    n164 = Multiply(x="Sin wave freq._y (Hz)", y=fxp<+/-,10,3> 2.0) -> (x*y=w418:fxp<+/-,41,9>)
    n165 = local read "Sin magnitude_y"() -> (w408:fxp<+/-,21,6>)
    n166 = local read "Sin magnitude_y"() -> (w401:fxp<+/-,21,6>)
    n167 = local read "Sin omega_y"() -> (w404:fxp<+/-,34,9>)
    n168 = Multiply(x=w418, y=w417) -> (x*y=w416:fxp<+/-,41,19>)
    n169 = Square(x=w404) -> (x^2=w403:fxp<+,34,18>)
    n170 = xnode "High Throughput Sine & Cosine"("x (pi)"=w416) -> ("sin(x)"=w398:fxp<+/-,16,2>, "cos(x)"=w406:fxp<+/-,16,2>)
    n171 = Multiply(x=w411, y=w410) -> (x*y=w409:fxp<+/-,34,9>)
    "Sin omega_y" <- w409
    n172 = Negate(x=w403) -> (-x=w402:fxp<+/-,35,19>)
    n173 = Multiply(x=w409, y=w408) -> (x*y=w407:fxp<+/-,33,15>)
    n174 = Multiply(x=w402, y=w401) -> (x*y=w400:fxp<+/-,34,20>)
    n175 = Multiply(x=w406, y=w407) -> (x*y=→"Dyr_sin_d":fxp<+/-,33,15>)
    n176 = Multiply(x="Sin magnitude_y", y=w398) -> (x*y=w414:fxp<+/-,37,8>)
    n177 = Multiply(x=w398, y=w400) -> (x*y=→"Dyr_sin_dd":fxp<+/-,35,20>)
    n178 = Add(x=w414, y="Sin offset_y") -> (x+y=→"Dyr_sin":fxp<+/-,37,8>)
    n179 = local read "Sin wave freq._p (Hz)"() -> (w375:fxp<+/-,32,6>)
    n180 = local read "Time now(s)"() -> (w393:fxp<+,52,14>)
    n181 = local read "Sin magnitude_p"() -> (w376:fxp<+/-,21,6>)
    n182 = local read "Sin magnitude_p"() -> (w378:fxp<+/-,21,6>)
    n183 = local read "Sin omega_p"() -> (w377:fxp<+/-,34,9>)
    n184 = Multiply(x="Sin wave freq._p (Hz)", y=fxp<+/-,10,3> 2.0) -> (x*y=w397:fxp<+/-,42,9>)
    n185 = Multiply(x=w397, y=w393) -> (x*y=w394:fxp<+/-,41,19>)
    n186 = Square(x=w377) -> (x^2=w389:fxp<+,34,18>)
    n187 = xnode "High Throughput Sine & Cosine"("x (pi)"=w394) -> ("sin(x)"=w380:fxp<+/-,16,2>, "cos(x)"=w385:fxp<+/-,16,2>)
    n188 = Multiply(x=w379, y=w375) -> (x*y=w392:fxp<+/-,34,9>)
    "Sin omega_p" <- w392
    n189 = Negate(x=w389) -> (-x=w388:fxp<+/-,35,19>)
    n190 = Multiply(x=w392, y=w376) -> (x*y=w391:fxp<+/-,33,15>)
    n191 = Multiply(x=w388, y=w378) -> (x*y=w387:fxp<+/-,35,19>)
    n192 = Multiply(x=w385, y=w391) -> (x*y=→"Dpr_sin_d":fxp<+/-,33,15>)
    n193 = Multiply(x=w380, y=w387) -> (x*y=→"Dpr_sin_dd":fxp<+/-,35,20>)
    n194 = Multiply(x="Sin magnitude_p", y=w380) -> (x*y=w383:fxp<+/-,37,8>)
    n195 = Add(x=w383, y="Sin offset_p") -> (x+y=→"Dpr_sin":fxp<+/-,37,8>)
  }
  n196 = while "Time reset" {
    shift-right: [w490] -> _
    shift-left: _ -> [w491]
    shift-right: [w485] -> _
    shift-left: _ -> [w486]
    stop <- FALSE stop-if-true
    n197 = local read "Stop motor_y"() -> (w492:bool)
    n198 = call "Tick Count3"() -> ("Tick Count(uSec)"=w490:u32)
    n199 = Subtract(x=w490, y=w491) -> (x-y=w489:u32)
    n200 = Add(x=w486, y=w489) -> (x+y=w488:u32)
    n201 = Select(t=u32 0, s=w492, f=w488) -> (s? t:f=w485:u32)
    n202 = To Fixed-Point(number=w485) -> (fixed-point=w484:fxp<+,32,32>)  [unwired: 1 in]
    n203 = Multiply(x=fxp<+,20,-18> 1.0000003385357559e-06, y=w484) -> (x*y=→"Time now(s)":fxp<+,52,14>)
  }
  n204 = while "Ini" {
    stop <- FALSE stop-if-true
    n205 = case shown="True" "Ini coe." {
      frame False {
      }
      frame True {
        w506 = i16 0 items=["Step", "Sine"] ("Command_p")
        w507 = i16 2 items=["Raw", "Avg.", "Avg. w. filter"] ("Strain selection_p")
        w508 = i16 0 items=["Step", "Sine"] ("Command_y")
        w509 = i16 2 items=["Raw", "Avg.", "Avg. w. filter"] ("Strain selection_y")
        w511 = fxp<+/-,25,-10> -5.851034075021744e-07  # S/F coeff_p
        w510 = fxp<+/-,25,-10> -1.0477961041033268e-06  # S/F coeff_y
        w517 = i16 0 items=["Backward", "Forward"] ("Drive mode")
        n206 = local write "Sin wave freq._y (Hz)"(fxp<+/-,32,6> 1.0 ("Sin wave freq. (Hz)")) -> ()
        n207 = local write "Sin magnitude_y"(fxp<+/-,22,7> 5.0 ("Sin magnitude")) -> ()
        n208 = local write "fy_tolorance"(fxp<+,22,6> 5.0 ("f_tolorance")) -> ()
        n209 = local write "Sin offset_y"(fxp<+/-,38,9> 0.0 ("Sin offset")) -> ()
        n210 = local write "Dyr_step"(fxp<+/-,22,7> 0.0 ("Dr")) -> ()
        n211 = local write "Kp_y"(fxp<+/-,36,9> 30.0 ("Kp")) -> ()
        n212 = local write "Kd_y"(fxp<+/-,36,9> 0.0 ("Kd")) -> ()
        n213 = local write "Kv_y"(fxp<+/-,22,8> 0.0 ("Kv")) -> ()
        n214 = local write "Bv_y"(fxp<+/-,22,8> 0.0 ("Bv")) -> ()
        n215 = local write "Ki_y"(fxp<+/-,36,9> 0.0 ("Ki")) -> ()
        n216 = local write "S/F coeff_p"(w511) -> ()
        n217 = local write "S/F coeff_y"(w510) -> ()
        n218 = local write "dFy_add"(FALSE ("dF_add")) -> ()
        n219 = local write "dFp_add"(FALSE ("dFp_add")) -> ()
        n220 = local write "Sin wave freq._p (Hz)"(fxp<+/-,32,6> 1.0 ("Sin wave freq._p (Hz)")) -> ()
        n221 = local write "Sin magnitude_p"(fxp<+/-,21,6> 5.0 ("Sin magnitude_p")) -> ()
        n222 = local write "fp_tolorance"(fxp<+,22,6> 5.0 ("fp_tolorance")) -> ()
        n223 = local write "Sin offset_p"(fxp<+/-,22,7> 0.0 ("Sin offset_p")) -> ()
        n224 = local write "Dpr_step"(fxp<+/-,22,7> 0.0 ("Dpr_step")) -> ()
        n225 = local write "Kp_p"(fxp<+/-,36,9> 30.0 ("Kp_p")) -> ()
        n226 = local write "Kd_p"(fxp<+/-,36,9> 0.0 ("Kd_p")) -> ()
        n227 = local write "Kv_p"(fxp<+/-,22,8> 0.0 ("Kv_p")) -> ()
        n228 = local write "Bv_p"(fxp<+/-,22,8> 0.0 ("Bv_p")) -> ()
        n229 = local write "Ki_p"(fxp<+/-,36,9> 0.0 ("Ki_p")) -> ()
        n230 = local write "Strain selection_p"(w507) -> ()
        n231 = local write "Strain selection_y"(w509) -> ()
        n232 = local write "Command_p"(w506) -> ()
        n233 = local write "Command_y"(w508) -> ()
        n234 = local write "Drive mode"(w517) -> ()
      }
    }
  }
  n235 = while "FIFO" {
    stop <- FALSE stop-if-true
    n236 = flat-sequence {
      frame #0 {
        n237 = call "Loop Timer"("Count(uSec)"=u32 1000) -> ()  [unwired: 1 out]
      }
      frame #1 {
        n238 = local read "D_y(mm)"() -> (w535:fxp<+/-,32,7>)
        n239 = local read "Raw Strain_y"() -> (w534:fxp<+/-,36,4>)
        n240 = local read "Strain_y (Avg)"() -> (w533:fxp<+/-,32,4>)
        n241 = local read "Strain_y (Avg w. f)"() -> (w532:fxp<+/-,36,8>)
        n242 = local read "D_p(mm)"() -> (w531:fxp<+/-,32,7>)
        n243 = local read "Raw Strain_p"() -> (w530:fxp<+/-,36,4>)
        n244 = local read "Strain_p (Avg)"() -> (w529:fxp<+/-,32,4>)
        n245 = local read "Strain_p (Avg w. f)"() -> (w526:fxp<+/-,36,8>)
        n246 = Build Array(w535, w534, w533, w532, w531, w530, w529, w526) -> (w528:fxp<+/-,40,8>[])
        n247 = xnode ("FIFO Write")("Element"=w528, "Timeout"=0) -> ()  [unwired: 1 in, 2 out]
      }
    }
  }
  n248 = while "PID force controller_y" {
    stop <- FALSE stop-if-true
    n249 = local read "Force_y"() -> (w553:fxp<+/-,32,10>)
    n250 = local read "fyt_d"() -> (w537:fxp<+/-,36,18>)
    n251 = local read "Fr_y"() -> (w539:fxp<+/-,32,10>)
    n252 = xnode "High Throughput Subtract"("x"=w539, "y"=w553) -> ("x-y"=w552:fxp<+/-,33,11>)
    "fy_tilde" <- w552
    n253 = Absolute Value(x=w552) -> (abs(x)=w543:fxp<+,33,11>)
    n254 = local read "fyt_i"() -> (w538:fxp<+/-,36,16>)
    n255 = xnode ("High Throughput Multiply")("x"="Kp_y", "y"=w552) -> ("x*y"=w550:fxp<+/-,64,20>)
    n256 = xnode ("High Throughput Multiply")("x"="Kd_y", "y"=w537) -> ("x*y"=w549:fxp<+/-,64,27>)
    n257 = xnode ("High Throughput Add")("x"=w550, "y"=w549) -> ("x+y"=w546:fxp<+/-,64,28>)
    n258 = xnode ("High Throughput Multiply")("x"="Ki_y", "y"=w538) -> ("x*y"=w547:fxp<+/-,64,25>)
    n259 = Greater?(x=w543, y="fy_tolorance") -> (0:w541:bool)
    n260 = xnode ("High Throughput Add")("x"=w546, "y"=w547) -> ("x+y"=w545:fxp<+/-,64,29>)
    n261 = Select(t=w545, s=w541, f=fxp<+/-,51,14> 0.0) -> (s? t:f=→"Fy_PID":fxp<+/-,64,29>)
  }
  n262 = while "Quadrature drive_p" {
    stop <- FALSE stop-if-true
    n263 = local read "dFp_PID"() -> (w556:fxp<+/-,36,18>)
    n264 = local read "omega_p (rad/s)"() -> (w562:fxp<+/-,20,9>)
    n265 = local read "Fp_PID"() -> (w557:fxp<+/-,36,16>)
    n266 = Select(t=w556, s="dFp_add", f=fxp<+,1,1> 0.0) -> (s? t:f=w560:fxp<+/-,36,18>)
    n267 = call "Oriental_step_motor_PKP225.vi"("F_Threshold"=fxp<+,12,12> 10.0, "dFmr"=w560, "omega"=w562, "Fmr"=w557) -> ("vq_F"=→"vq_p_F":fxp<+/-,20,5>, "vd_F"=→"vd_p_F":fxp<+/-,20,5>)  [unwired: 6 in]
  }
  n268 = while "PID force controller_p" {
    stop <- FALSE stop-if-true
    n269 = local read "Force_p"() -> (w577:fxp<+/-,32,10>)
    n270 = local read "fpt_d"() -> (w568:fxp<+/-,36,18>)
    n271 = local read "Fr_p"() -> (w578:fxp<+/-,32,10>)
    n272 = xnode "High Throughput Subtract"("x"=w578, "y"=w577) -> ("x-y"=w569:fxp<+/-,33,11>)
    "fp_tilde" <- w569
    n273 = local read "fpt_i"() -> (w566:fxp<+/-,34,18>)
    n274 = xnode ("High Throughput Multiply")("x"="Kp_p", "y"=w569) -> ("x*y"=w567:fxp<+/-,64,20>)
    n275 = xnode ("High Throughput Multiply")("x"="Kd_p", "y"=w568) -> ("x*y"=w583:fxp<+/-,64,27>)
    n276 = Absolute Value(x=w569) -> (abs(x)=w576:fxp<+,33,11>)
    n277 = xnode ("High Throughput Add")("x"=w567, "y"=w583) -> ("x+y"=w581:fxp<+/-,64,28>)
    n278 = xnode ("High Throughput Multiply")("x"="Ki_p", "y"=w566) -> ("x*y"=w582:fxp<+/-,64,27>)
    n279 = xnode ("High Throughput Add")("x"=w581, "y"=w582) -> ("x+y"=w572:fxp<+/-,64,29>)
    n280 = Greater?(x=w576, y="fp_tolorance") -> (0:w573:bool)
    n281 = Select(t=w572, s=w573, f=fxp<+,1,1> 0.0) -> (s? t:f=→"Fp_PID":fxp<+/-,64,29>)
  }
  n282 = while "PD position controller_p" {
    stop <- FALSE stop-if-true
    n283 = local read "Drive mode"() -> (w586:i16)
    n284 = case shown="1" w586 {
      tunnel: [fxp<+/-,62,19> 0.0 w589] -> w585
      frame 0, Default {
        # "Backward"
      }
      frame 1 {
        # "Forward"
        n285 = local read "D_p(mm)"() -> (w596:fxp<+/-,32,7>)
        n286 = local read "Dp_error_d"() -> (w588:fxp<+/-,33,8>)
        n287 = local read "Dpr_for"() -> (w595:fxp<+/-,22,7>)
        n288 = Subtract(x=w595, y=w596) -> (x-y=w594:fxp<+/-,24,8>)
        "Dp_error" <- w594
        n289 = Multiply(x=w594, y="Kv_p") -> (x*y=w591:fxp<+/-,34,16>)
        n290 = Multiply(x=w588, y="Bv_p") -> (x*y=w590:fxp<+/-,55,16>)
        n291 = Add(x=w591, y=w590) -> (x+y=w589:fxp<+/-,56,17>)
      }
    }
    "Fr_p" <- w585
  }
  n292 = while "All switch" {
    stop <- FALSE stop-if-true
    n293 = case shown="False" "Encoder reset" {
      frame False {
        n294 = local write "Encoder reset_p"(FALSE ("Encoder reset_p")) -> ()
        n295 = local write "Encoder reset_y"(FALSE ("Encoder reset_y")) -> ()
      }
      frame True {
        n296 = local write "Encoder reset_p"(TRUE ("Encoder reset_p")) -> ()
        n297 = local write "Encoder reset_y"(TRUE ("Encoder reset_y")) -> ()
      }
    }
  }
  n298 = while "Derivative" {
    stop <- FALSE stop-if-true
    n299 = local read "Dpr_sin_dd"() -> (w611:fxp<+/-,35,20>)
    n300 = local read "Stop motor_y"() -> (w617:bool)
    n301 = local read "Dyr_sin_dd"() -> (w619:fxp<+/-,35,20>)
    n302 = local read "Dpr_sin_d"() -> (w613:fxp<+/-,33,15>)
    n303 = local read "Stop motor_p"() -> (w609:bool)
    n304 = local read "Dyr_sin_d"() -> (w622:fxp<+/-,33,15>)
    n305 = local read "Dp_error"() -> (w614:fxp<+/-,22,7>)
    n306 = local read "Dy_error"() -> (w623:fxp<+/-,22,7>)
    n307 = local read "Dp_dd"() -> (w612:fxp<+/-,36,25>)
    n308 = local read "Dy_dd"() -> (w620:fxp<+/-,36,25>)
    n309 = Subtract(x=w622, y=w623) -> (x-y=w621:fxp<+/-,34,16>)
    n310 = Subtract(x=w619, y=w620) -> (x-y=w618:fxp<+/-,41,26>)
    n311 = Subtract(x=w613, y=w614) -> (x-y=w606:fxp<+/-,34,16>)
    n312 = Subtract(x=w611, y=w612) -> (x-y=w610:fxp<+/-,41,26>)
    n313 = Select(t=fxp<+,1,1> 0.0, s=w617, f=w621) -> (s? t:f=→"Dy_error_d":fxp<+/-,34,16>)
    n314 = Select(t=fxp<+/-,64,49> 0.0, s=w617, f=w618) -> (s? t:f=→"Dy_error_dd":fxp<+/-,64,49>)
    n315 = Select(t=fxp<+,1,1> 0.0, s=w609, f=w606) -> (s? t:f=→"Dp_error_d":fxp<+/-,34,16>)
    n316 = Select(t=fxp<+/-,41,26> 0.0, s=w609, f=w610) -> (s? t:f=→"Dp_error_dd":fxp<+/-,41,26>)
  }
  n317 = while "ft_d" {
    stop <- FALSE stop-if-true
    n318 = local read "Dy_error_dd"() -> (w641:fxp<+/-,36,16>)
    n319 = local read "Dp_error_dd"() -> (w632:fxp<+/-,36,16>)
    n320 = local read "Dy_error_d"() -> (w643:fxp<+/-,33,8>)
    n321 = local read "Dp_error_d"() -> (w634:fxp<+/-,33,8>)
    n322 = local read "Kv_p"() -> (w635:fxp<+/-,22,8>)
    n323 = local read "Bv_p"() -> (w633:fxp<+/-,22,8>)
    n324 = local read "Kv_y"() -> (w644:fxp<+/-,22,8>)
    n325 = local read "Bv_y"() -> (w642:fxp<+/-,22,8>)
    n326 = local read "Force_y"() -> (w637:fxp<+/-,32,10>)
    n327 = Multiply(x=w643, y=w644) -> (x*y=w639:fxp<+/-,55,16>)
    n328 = Multiply(x=w641, y=w642) -> (x*y=w640:fxp<+/-,58,24>)
    n329 = Multiply(x=w634, y=w635) -> (x*y=w630:fxp<+/-,55,16>)
    n330 = Multiply(x=w632, y=w633) -> (x*y=w631:fxp<+/-,58,24>)
    n331 = local read "Force_p"() -> (w628:fxp<+/-,32,10>)
    n332 = Add(x=w639, y=w640) -> (x+y=w638:fxp<+/-,63,24>)
    n333 = Add(x=w630, y=w631) -> (x+y=w629:fxp<+/-,63,24>)
    n334 = Subtract(x=w638, y=w637) -> (x-y=→"fyt_d":fxp<+/-,63,24>)
    n335 = Subtract(x=w629, y=w628) -> (x-y=→"fpt_d":fxp<+/-,63,24>)
  }
  n336 = while "Encoder_p" {
    shift-right: [w655] -> _
    shift-left: _ -> [w656]
    shift-right: [w657] -> _
    shift-left: _ -> [w658]
    shift-right: [w651] -> _
    shift-left: _ -> [w659]
    stop <- FALSE stop-if-true
    w648 = fxp<+/-,32,0> 0.0020454544574022293  # L*(18/22)/800
    n337 = xnode "FPGA I/O Node"() -> ("Mod4/DI0"=w653:bool, "Mod4/DI1"=w654:bool)  [unwired: 2 in, 2 out]
    n338 = call "encoder_sub.vi"("A_pre"=w656, "B_pre"=w658, "Encoder Position_pre"=w659, "A input"=w653, "Encoder Position Reset"="Encoder reset_p", "B input"=w654) -> ("A"=w655:bool, "B"=w657:bool, "Encoder Position (Counts)"=w651:i32)  [unwired: 19 in]
    "Encoder Position_p" <- w651
    n339 = To Fixed-Point(number=w651) -> (fixed-point=w650:fxp<+/-,32,32>)  [unwired: 1 in]
    n340 = xnode ("High Throughput Multiply")("x"=w650, "y"=w648) -> ("x*y"=→"D_p(mm)":fxp<+/-,64,32>)
    n341 = xnode ("High Throughput Multiply")("x"=w650, "y"=fxp<+/-,16,1> 0.125) -> ("x*y"=→"rad_p(NrTheta)":fxp<+/-,48,33>)
  }
  n342 = while "Omega_p(T method)" {
    shift-right: [w671] -> _
    shift-left: _ -> [w669]
    shift-right: [w664] -> _
    shift-left: _ -> [w670]
    shift-right: [w666] -> _
    shift-left: _ -> [w668]
    stop <- FALSE stop-if-true
    w663 = fxp<+/-,32,0> 0.2604353614151478  # L/2/pi*(18/22)
    n343 = local read "Encoder Position_p"() -> (w671:i32)
    n344 = call "Tick Count4"() -> ("Tick Count(Ticks)"=w667:u32)
    n345 = call "omega_sub_Encoder_800ppr.vi"("mt0"="mt0_omega_p", "omega_pre"=w670, "ticks_m_pre"=w668, "ticks"=w667, "count_pre"=w669, "count"=w671) -> ("ticks_m"=w666:u32, "mt"=→"mt_omega_p":u32, "omega"=w664:fxp<+/-,36,13>)  [unwired: 3 in]
    "omega_p (rad/s)" <- w664
    n346 = xnode ("High Throughput Multiply")("x"=w663, "y"=w664) -> ("x*y"=→"Dp_d (mm/s)":fxp<+/-,64,13>)
  }
  n347 = xnode "FPGA I/O Node"("error in"=w1, "Mod6/Stop"=TRUE) -> ()  [unwired: 1 in, 2 out]
